vi "Next Step.vi"(8 "error in (no error)":errorcluster, 11 "Varian Magnet Scan in":refnum<class "Varian Magnet Scan.lvclass">) -> (0 "error out":errorcluster, 1 "Current Step":u32, 2 "Current Position":dbl, 3 "Varian Magnet Scan out":refnum<class "Varian Magnet Scan.lvclass">)   [LabVIEW 2009, in "Varian Magnet Scan.lvclass"]
uses:
  Varian Magnet Scan.lvclass
  Scanner/Scanner.lvclass
  Instruments/Varian Magnet/Varian Magnet.lvclass
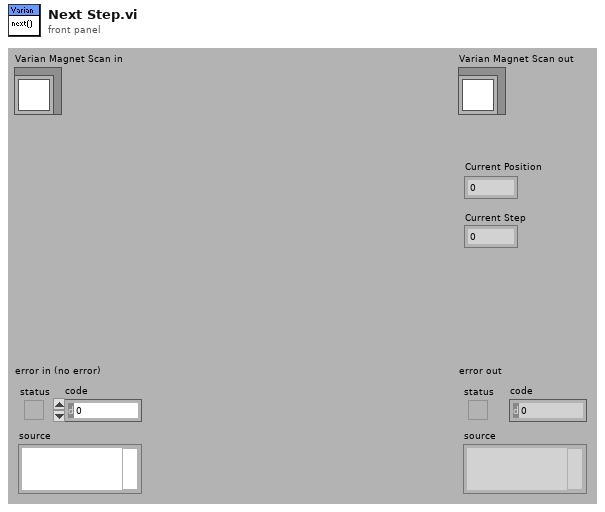
[diagram p1: front panel]
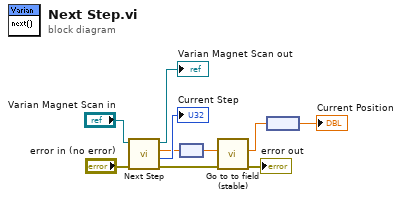
[diagram p0: block diagram]
diagram:
  n1 = call-parent "Next Step.vi"("error in (no error)"="error in (no error)", "Scanner in"="Varian Magnet Scan in") -> ("error out"=w2:errorcluster, "Current Step"=→"Current Step":u32, "Current Position"=w6:dbl, "Scanner out"=→"Varian Magnet Scan out":refnum<class "Varian Magnet Scan.lvclass">)  [unwired: 6 out]
  n2 = node(w6) -> (w4:dbl[unit])
  n3 = call "Go to to field (stable).vi"("error in"=w2, "Desired field"=w4) -> ("error out"=→"error out":errorcluster, "Current field"=w5:dbl[unit])  [unwired: 8 out]
  n4 = node(w5) -> (→"Current Position":dbl)
